vi "Init.vi"(5 "Required Scope(s)":string[](array[string]), 7 "Redirect URL (http://localhost)":string, 10 "Token URL":string, 11 "Auth URL":string) -> (3 "Request out":refnum<class "Request.lvclass">)   [LabVIEW 2020, in "OAuth2.lvlib" / "Request.lvclass"]
doc: "Configures the OAuth2 Request. The details for these values are determined / configured with the authorization provider.\n\nThe Scopes input is optional to allow easier reuse of a configured Request instance with different needed scopes but scopes must be defined either directly on the Request or when initiating the OAuth2 authorization request.\n\nUnless there is a need to use a specific listening port, the Redirect URL can usually be left blank. Leaving the Redirect URL blank allows the application to receive the redirect request from the browser that the authorization specifies and without a port specified allows the OS to specify a random port number that will be used."
uses:
  Request.lvclass
  Request.lvclass/Request.ctl
  lv-stream/stream/URI/URI.lvclass
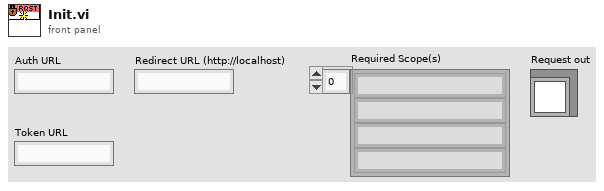
[diagram p1: front panel]
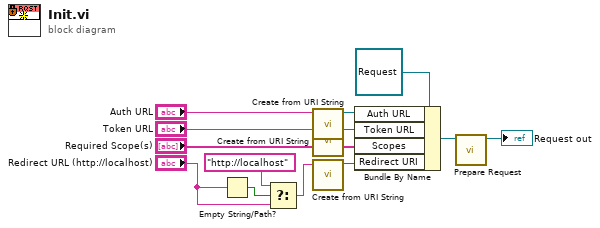
[diagram p0: block diagram]
diagram:
  n1 = Empty String/Path?(string/path="Redirect URL (http://localhost)") -> (empty?=w11:bool)
  n2 = Select(t="http://localhost", s=w11, f="Redirect URL (http://localhost)") -> (s? t:f=w9:string)
  n3 = call "Create from URI String.vi"("URI String"="Auth URL") -> ("URI out"=w13:refnum<class "URI.lvclass">)  [unwired: 9 in, 1 out]
  n4 = call "Create from URI String.vi"("URI String"="Token URL") -> ("URI out"=w12:refnum<class "URI.lvclass">)  [unwired: 9 in, 1 out]
  n5 = call "Create from URI String.vi"("URI String"=w9) -> ("URI out"=w8:refnum<class "URI.lvclass">)  [unwired: 9 in, 1 out]
  n6 = Bundle By Name(cluster=refnum<class "Request.lvclass"> refnum ("Request out"), "Auth URL"=w13, "Token URL"=w12, "Scopes"="Required Scope(s)", "Redirect URI"=w8) -> (w7:refnum<class "Request.lvclass">)
  n7 = call "Prepare Request.vi"("Request in"=w7) -> ("Request out"=→"Request out":refnum<class "Request.lvclass">)  [unwired: 10 in]
